vi "pp2_util_addToMean.vi"(8 "New value":dbl=7.0, 10 "Original count":i64=1, 11 "Original mean":dbl=3.0) -> (3 "New mean":dbl)   [LabVIEW 2013]
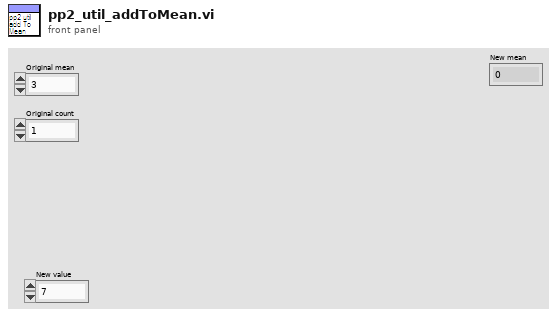
[diagram p1: front panel]
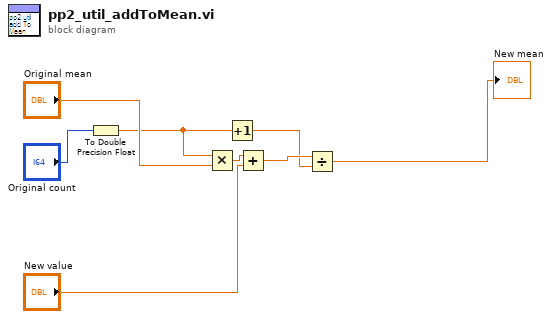
[diagram p0: block diagram]
diagram:
  n1 = To Double Precision Float(number="Original count") -> (double precision float=w2:dbl)
  n2 = Multiply(x=w2, y="Original mean") -> (x*y=w8:dbl)
  n3 = Increment(x=w2) -> (x+1=w1:dbl)
  n4 = Add(x=w8, y="New value") -> (x+y=w7:dbl)
  n5 = Divide(x=w7, y=w1) -> (x/y=→"New mean":dbl)
